vi "CRYLimit Table Insert.vi"(11 "Limit Table":refnum<vi>) -> ()   [LabVIEW 2013]
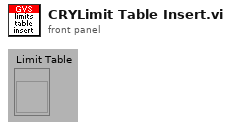
[diagram p1: front panel]
types:
  T1 = typedef "LVRowAndColumnTypeDef.ctl" = cluster{"Row":i32, "Column":i32}
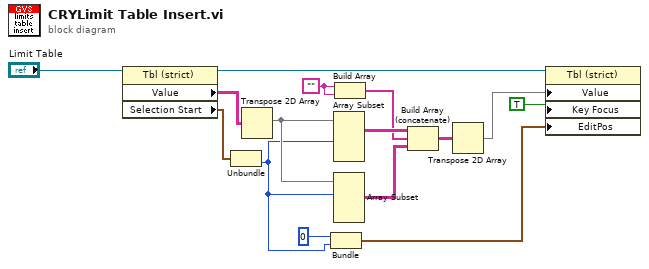
[diagram p0: block diagram]
diagram:
  w13 = ""
  n1 = property class="Tbl (strict)"(reference="Limit Table") -> (reference out=w4:refnum<vi>, "Value"=w9:string[][], "Selection Start"=w7:T1)  [unwired: 1 in, 1 out]
  n2 = Unbundle(w7) -> ("Column"=w5:i32)  [unwired: 1 out]
  n3 = Transpose 2D Array(2D array=w9) -> (transposed array=w14:string[][])
  n4 = Bundle(0, "Column"=w5) -> (w1:cluster{i32, "Column":i32})  [unwired: 1 out]
  n5 = Array Subset(array=w14, length (row)=w5) -> (w12:string[][])  [unwired: 3 in]
  n6 = Array Subset(array=w14, index (row)=w5) -> (w11:string[][])  [unwired: 3 in]
  n7 = Build Array(w13, w13) -> (w10:string[])
  n8 = Build Array (concatenate)(w12, w10, w11) -> (w6:string[][])
  n9 = Transpose 2D Array(2D array=w6) -> (transposed array=w3:string[][])
  n10 = property class="Tbl (strict)"(reference=w4, "Value"=w3, "Key Focus"=TRUE ("Write Attribute"), "EditPos"=w1) -> ()  [unwired: 1 in, 2 out]
